vi "Clear.vi"(8 "error in (no error)":errorcluster caption="错误输入（无错误）", 11 "Queue 输入":refnum<class "Queue.lvclass"> caption="DNL_LabVIEW Object in") -> (0 "error out":errorcluster caption="错误输出", 3 "Queue 输出":refnum<class "Queue.lvclass"> caption="DNL_LabVIEW Object out")   [LabVIEW 2012, in "Queue.lvclass"]
uses:
  Queue.lvclass
  Queue.lvclass/Queue.ctl
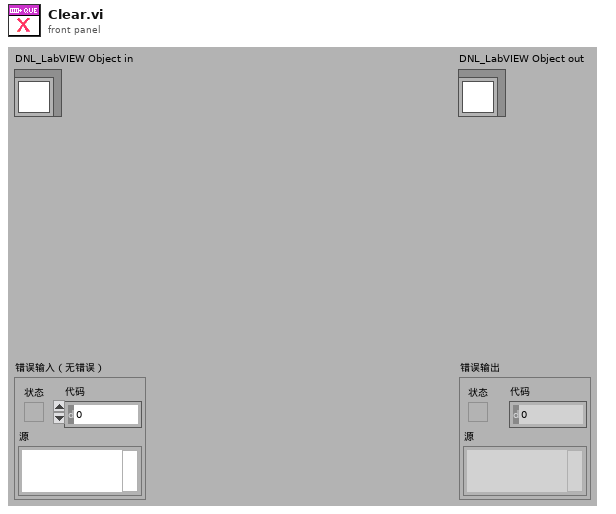
[diagram p1: front panel]
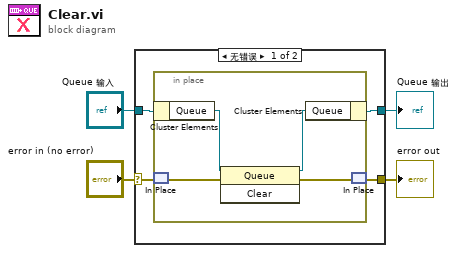
[diagram p0: block diagram]
diagram:
  n1 = case shown="无错误" "error in (no error)" {
    selector: "error in (no error)" -> [w6 w14]
    tunnel: [w5 w14] -> w3
    tunnel: [w7 w13] -> w1
    tunnel: "Queue 输入" -> [w8 w13]
    frame No Error {
      n2 = in-place {
        n3 = in-place-cluster #1(w8) -> ("Queue"=w12:refnum<k24>)
        n4 = in-place-match #2(w6) -> (w9:errorcluster)
        n5 = invoke class="Queue" method="Clear"(reference=w12, error in=w9) -> (reference out=w11:refnum<k24>, error out=w10:errorcluster)  [unwired: 1 in, 1 out]
        n6 = in-place-cluster #1("Queue"=w11) -> (w7:refnum<class "Queue.lvclass">)
        n7 = in-place-match #2(w10) -> (w5:errorcluster)
      }
    }
    frame Error {
    }
  }
  "error out" <- w3
  "Queue 输出" <- w1
